vi "Replace Placeholder VI with Method VI.vi"(8 "error in (no error)":errorcluster, 10 "Method VI Path":path, 11 "DVR VI Path":path) -> (0 "error out":errorcluster)   [LabVIEW 2016, in "SLL Class DVR API Generator.lvlib"]
uses:
  SLL Class DVR API Generator.lvlib
  <vilib>/Utility/traverseref.llb/TRef TravTarget.ctl
  <vilib>/Utility/traverseref.llb/VI Scripting - Traverse.lvlib
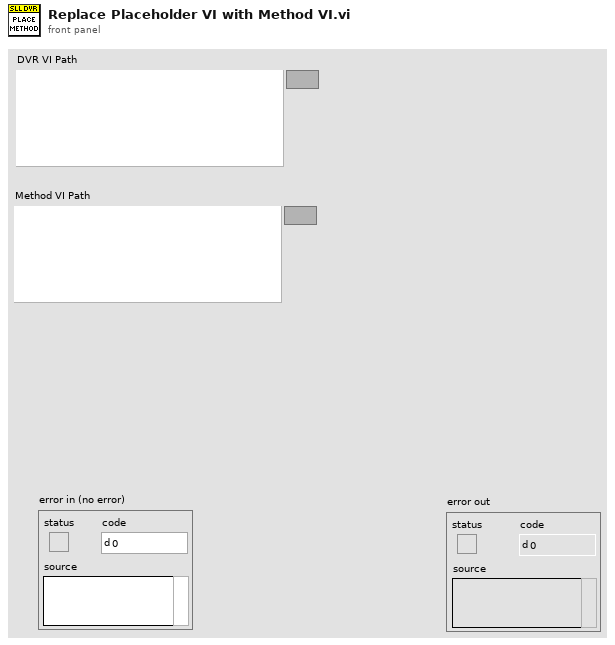
[diagram p1: front panel]
types:
  T1 = typedef "TRef TravTarget.ctl" = enum16{"FP", "BD", "Other"}
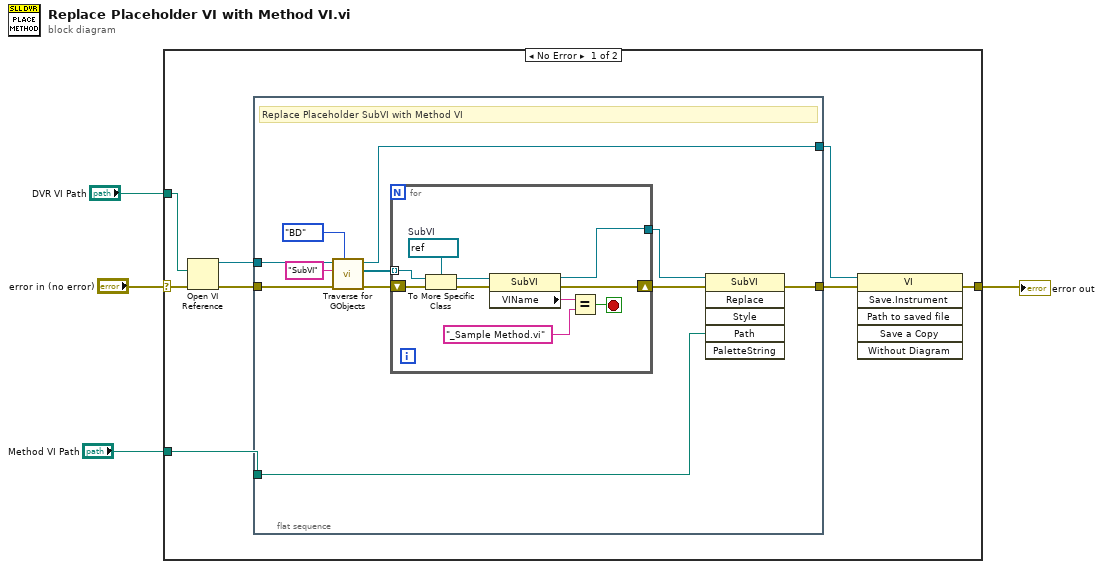
[diagram p0: block diagram]
diagram:
  n1 = case shown="No Error" "error in (no error)" {
    selector: "error in (no error)" -> [w12 w34]
    tunnel: [w10 w34] -> w3
    tunnel: "DVR VI Path" -> [w11 _]
    tunnel: "Method VI Path" -> [w7 _]
    frame No Error {
      n2 = Open VI Reference(vi path=w11, error in (no error)=w12) -> (vi reference=w9:refnum<vi>, error out=w8:errorcluster)  [unwired: 4 in]
      n3 = flat-sequence {
        tunnel: w9 -> [w23]
        tunnel: w8 -> [w20]
        tunnel: [w16] -> w6
        tunnel: w7 -> [w14]
        tunnel: [w13] -> w5
        frame #0 {
          # "Replace Placeholder SubVI with Method VI"
          n4 = call <vilib>:"Traverse for GObjects.vi"("Traverse Target"=TRef_TravTarget."BD", "error in (no error)"=w20, "Class Name"="SubVI", "VI Refnum"=w23) -> ("error out"=w19:errorcluster, "References"=w17:refnum<vi>[], "dup VI Refnum"=w13:refnum<vi>)  [unwired: 4 in, 1 out]
          n5 = for {
            shift-right: [w29] -> w18
            shift-left: w19 -> [w33]
            tunnel: w17 -> [w31] mode=indexing
            tunnel: [w24] -> w15
            stop <- w25 stop-if-true
            w30 = refnum<vi> refnum  # SubVI
            n6 = To More Specific Class(target class=w30, reference=w31, error in=w33) -> (specific class reference=w28:refnum<vi>, error out=w32:errorcluster)
            n7 = property class="SubVI"(reference=w28, error in=w32) -> (reference out=w24:refnum<vi>, error out=w29:errorcluster, "VIName"=w27:string)
            n8 = Equal?(x=w27, y="_Sample Method.vi") -> (x = y?=w25:bool)
          }
          n9 = invoke class="SubVI" method="Replace"(reference=w15, error in=w18, "Path"=w14) -> (error out=w16:errorcluster)  [unwired: 3 in, 5 out]
        }
      }
      n10 = invoke class="VI" method="Save.Instrument"(reference=w5, error in=w6) -> (error out=w10:errorcluster)  [unwired: 4 in, 5 out]
    }
    frame Error {
    }
  }
  "error out" <- w3
